vi "exportGraphsToPDF.Strings.vi"(7 "Red":refnum<vi>, 8 "error in (no error)":errorcluster, 9 "Input Cluster":cluster{dbl, dbl, dbl, dbl}, 10 "Blue":refnum<vi>, 11 "PDF Report duplicate":T21) -> (0 "error out":errorcluster, 3 "PDF Report OUT":T21)   [LabVIEW 2013, in "main.lvlib"]
uses:
  main.lvlib
  C:/Program Files (x86)/National Instruments/LabVIEW 2013/user.lib/Exaprom PDF/DLL/itextsharp.dll
  Program Files (x86)/National Instruments/LabVIEW 2013/user.lib/Exaprom PDF/DLL/itextsharp.dll
  <userlib>/Exaprom PDF/Controls/Font cluster.ctl
  <userlib>/Exaprom PDF/Controls/Font size.ctl
  <userlib>/Exaprom PDF/Controls/Font color.ctl
  <userlib>/Exaprom PDF/Controls/Unit.ctl
  <userlib>/Exaprom PDF/Controls/Paragraphe cluster.ctl
  <userlib>/Exaprom PDF/Controls/Texte alignement.ctl
  <userlib>/Exaprom PDF/Controls/Line spacing.ctl
  <userlib>/Exaprom PDF/Controls/Page dimensions.ctl
  <userlib>/Exaprom PDF/Controls/Page Orientation.ctl
  <userlib>/Exaprom PDF/Controls/Image or Table Caption.ctl
  <userlib>/Exaprom PDF/Controls/Header Footer [ ].ctl
  <userlib>/Exaprom PDF/Controls/Header Footer cluster.ctl
  <userlib>/Exaprom PDF/Controls/Header Footer Type.ctl
  <userlib>/Exaprom PDF/Controls/Header footer horiz alignment.ctl
  <userlib>/Exaprom PDF/Controls/Cell Vertical alignment.ctl
  <userlib>/Exaprom PDF/Controls/Page number.ctl
  <userlib>/Exaprom PDF/Controls/Header Footer Line.ctl
  <userlib>/Exaprom PDF/Controls/Watermark cluster2.ctl
  <userlib>/Exaprom PDF/Controls/Watermark Position.ctl
  <userlib>/Exaprom PDF/Controls/System Fonts.ctl
  <userlib>/Exaprom PDF/VIs/Text/Append Paragraph.vi
panel:
  # "X"
  # "Y"
  # "X"
  # "Y"
  # "X"
  # "Y"
  # "X"
  # "Y"
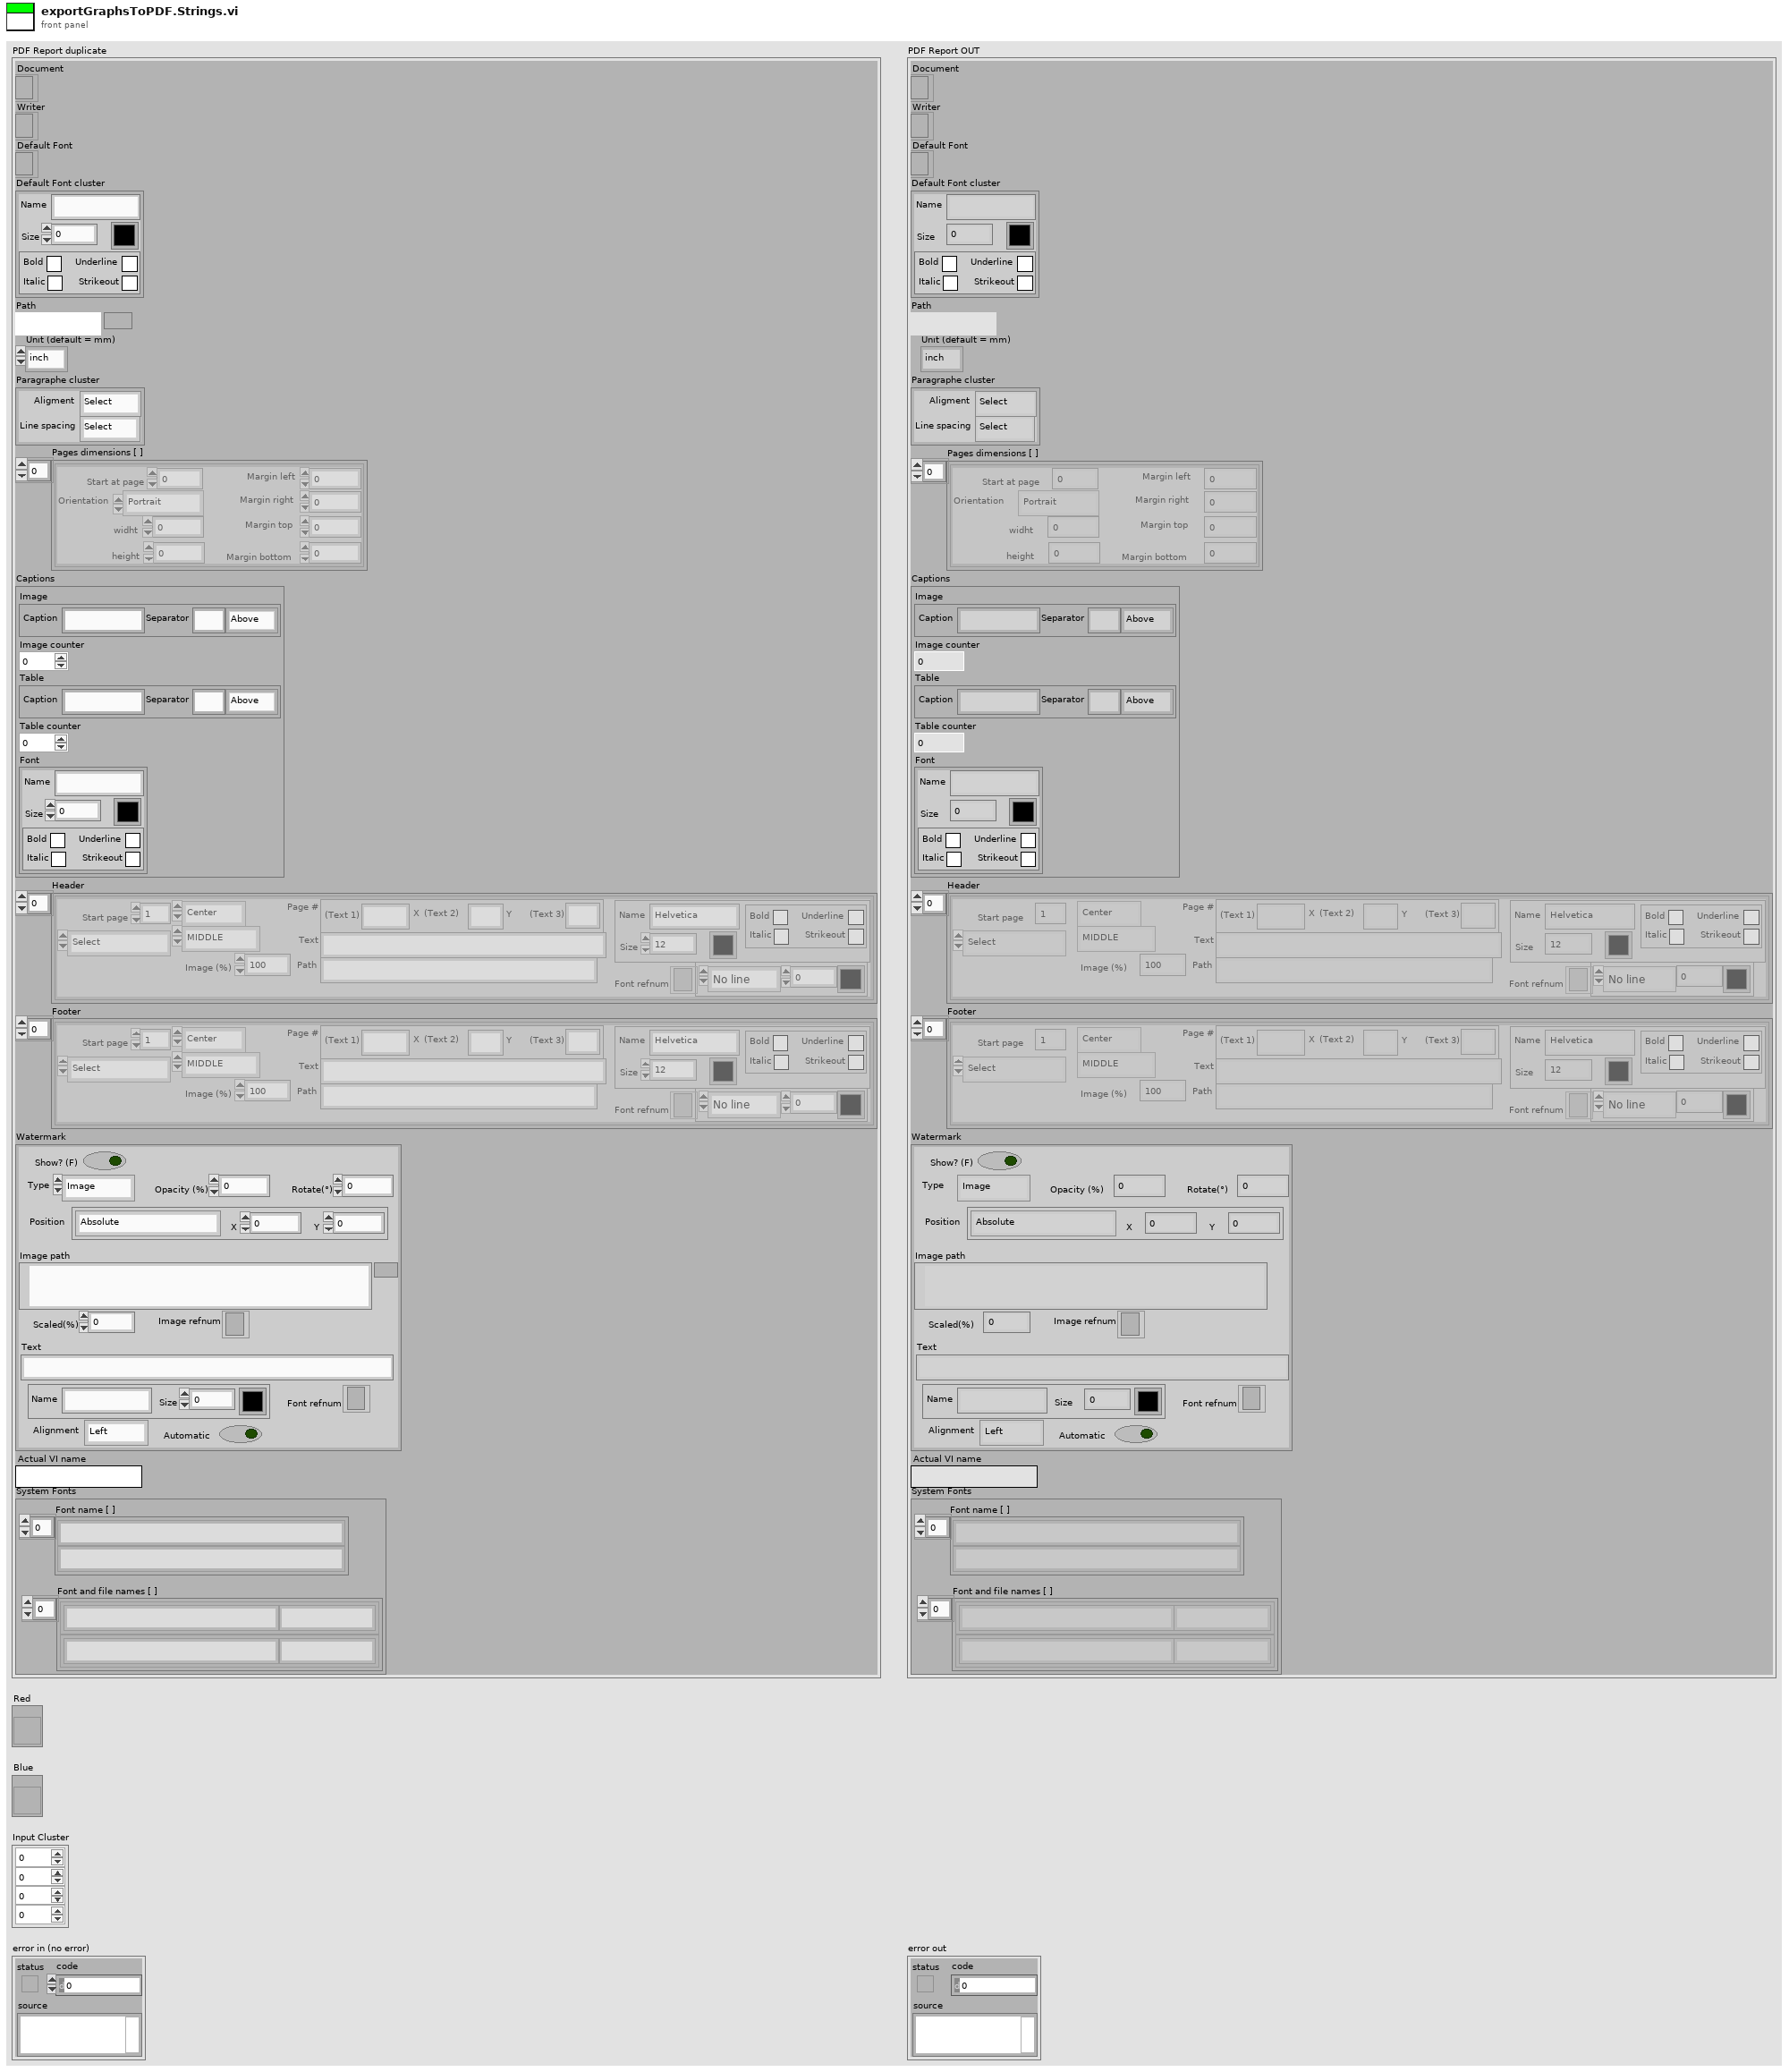
[diagram p1: front panel]
types:
  T1 = typedef "Font cluster.ctl" = cluster{"Name":string, "Size":T2, "Color":T3, "Style":cluster{"Bold":bool, "Italic":bool, "Underline":bool, "Strikeout":bool}}
  T2 = typedef "Font size.ctl" = sgl
  T3 = typedef "Font color.ctl" = u32
  T4 = typedef "Unit.ctl" = enum16{"inch", "mm"}
  T5 = typedef "Paragraphe cluster.ctl" = cluster{" Aligment":T6, "Line spacing":T7}
  T6 = typedef "Texte alignement.ctl" = enum16{"Select", "CENTER", "JUSTIFY", "LEFT", "RIGHT"}
  T7 = typedef "Line spacing.ctl" = enum16{"Select", "1.0", "1.5", "2.0"}
  T8 = typedef "Page dimensions.ctl" = cluster{"Start at page":i32, "Orientation":T9, "widht":sgl, "height":sgl, "Margin left":sgl, "Margin right":sgl, "Margin top":sgl, "Margin bottom":sgl}
  T9 = typedef "Page Orientation.ctl" = enum16{"Portrait", "Landscape"}
  T10 = typedef "Image or Table Caption.ctl" = cluster{"Caption":string, "Separator":string, "Position":enum16{"Above", "Below"}}
  T11 = typedef "Header Footer [ ].ctl" = T12[]
  T12 = typedef "Header Footer cluster.ctl" = cluster{"Start page":i32, "Type":T13, "Alignment":T14, "Vertical Alignement":T15, "Image (%)":sgl, "Page #":T16, "Text":string, "Path":string, "Font":T1, "Font refnum":refnum<k24>, "Line":cluster{"Line":T17, "Thickness (points)":sgl, "Colour":T3}}
  T13 = typedef "Header Footer Type.ctl" = enum16{"Select", "Text", "Text + hyperlink", "Page number", "Image", "Image + hyperlink"}
  T14 = typedef "Header footer horiz alignment.ctl" = enum16{"Left", "Center", "Right"}
  T15 = typedef "Cell Vertical alignment.ctl" = enum16{"TOP", "MIDDLE", "BOTTOM"}
  T16 = typedef "Page number.ctl" = cluster{"Text 1":string, "Text 2":string, "Text 3":string}
  T17 = typedef "Header Footer Line.ctl" = enum16{"No line", "Horizontal line"}
  T18 = typedef "Watermark cluster2.ctl" = cluster{"Show? (F)":bool, "Type":enum16{"Image", "Text"}, "Opacity (%)":sgl, "Rotate(°)":sgl, "Position":cluster{"Position":T19, "X":sgl, "Y":sgl}, "Image path":path, "Scaled(%)":sgl, "Image refnum":refnum<k24>, "Text":string, "Font":cluster{"Name":string, "Size":T2, "Color":T3}, "Font refnum":refnum<k24>, "Alignment":T14, "Automatic":bool}
  T19 = typedef "Watermark Position.ctl" = enum16{"Absolute", "Center (page)", "Center (text section)"}
  T20 = typedef "System Fonts.ctl" = cluster{"Font name [ ]":string[], "Font and file names [ ]":cluster{"Font name":string, "File name":string}[]}
  T21 = cluster{"Document":refnum<k24>, "Writer":refnum<k24>, "Default Font":refnum<k24>, "Default Font cluster":T1, "Path":path, "Unit (default = mm)":T4, "Paragraphe cluster":T5, "Pages dimensions [ ]":T8[], "Captions":cluster{"Image":T10, "Image counter":u16, "Table":T10, "Table counter":u16, "Font":T1}, "Header":T11, "Footer":T11, "Watermark ":T18, "Actual VI name":string, "System Fonts":T20}
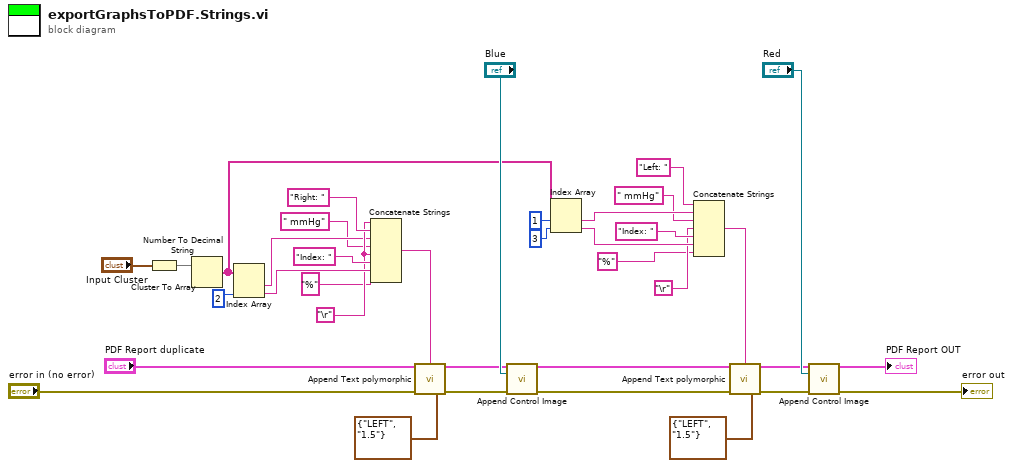
[diagram p0: block diagram]
diagram:
  w7 = "\r"
  n1 = Cluster To Array(cluster="Input Cluster") -> (array=w25:dbl[])
  n2 = Number To Decimal String(number=w25) -> (decimal integer string=w18:string[])  [unwired: 1 in]
  n3 = Index Array(array=w18, index #2=2 ("index")) -> (element #1=w3:string, element #2=w23:string)  [unwired: 1 in]
  n4 = Concatenate Strings(w7, "Right: ", w3, " mmHg" ("string"), w7, "Index: " ("string"), w23, "%") -> (w29:string)
  n5 = call-poly <userlib>:"Append Text polymorphic.vi"("PDF Report"="PDF Report duplicate", "Text"=w29, "error in (no error)"="error in (no error)", "Paragraph properties"=T5 {" Aligment"=enum."LEFT", "Line spacing"=enum."1.5"}) -> ("PDF Report duplicate"=w31:T21, "error out"=w32:errorcluster)  [unwired: 10 in]
  n6 = call <userlib>:"Append Control Image.vi"("PDF Report IN"=w31, "Ctrl reference"="Blue", "error in (no error)"=w32) -> ("PDF Report OUT"=w14:T21, "error out"=w15:errorcluster)  [unwired: 11 in]
  n7 = Index Array(array=w18, index #1=1 ("index"), index #2=3 ("index")) -> (element #1=w20:string, element #2=w19:string)
  n8 = Concatenate Strings("Left: ", w20, " mmHg" ("string"), "\r", "Index: " ("string"), w19, "%") -> (w13:string)
  n9 = call-poly <userlib>:"Append Text polymorphic.vi"("PDF Report"=w14, "Text"=w13, "error in (no error)"=w15, "Paragraph properties"=T5 {" Aligment"=enum."LEFT", "Line spacing"=enum."1.5"}) -> ("PDF Report duplicate"=w17:T21, "error out"=w16:errorcluster)  [unwired: 10 in]
  n10 = call <userlib>:"Append Control Image.vi"("PDF Report IN"=w17, "Ctrl reference"="Red", "error in (no error)"=w16) -> ("PDF Report OUT"=→"PDF Report OUT":T21, "error out"=→"error out":errorcluster)  [unwired: 11 in]
